vi "Main.vi"() -> ()   [LabVIEW 2023]
uses:
  Ctl/QMH Fundamentals - Message Cluster.ctl
  Ctl/Command.ctl
  Ctl/Global Parameter.ctl
  e830df23-c5e2-412d-a348-f1522410b5be.vi
  System.Speech
  3f4bac93-3011-4ff6-ad61-7a3954b40021.vi
panel:
  out "当前状态":string
  in  "Start?":bool
  out "识别结果 2":string caption="识别结果"
  out "灯 2":bool
  out "系统回复 2":string
  out "命令列表 2":string[](array[string])=["你好", "早上好", "中午好", "下午好", "分析", "测试", "音乐", "开灯", "关灯", "再见"] caption="命令列表"
  out "当前用户 2":string caption="当前用户"
  in  "LogOut 2":bool
  out "当前用户":string
  in  "LogOut":bool
  out "命令列表":string[](array[string])=["你好", "早上好", "中午好", "下午好", "分析", "测试", "音乐", "开灯", "关灯", "再见"]
  out "灯":bool
  out "系统回复":string
  out "识别结果":string
  # "基于声卡的语音识别与音频分析系统"
  # "基于声卡的语音识别与音频分析系统"
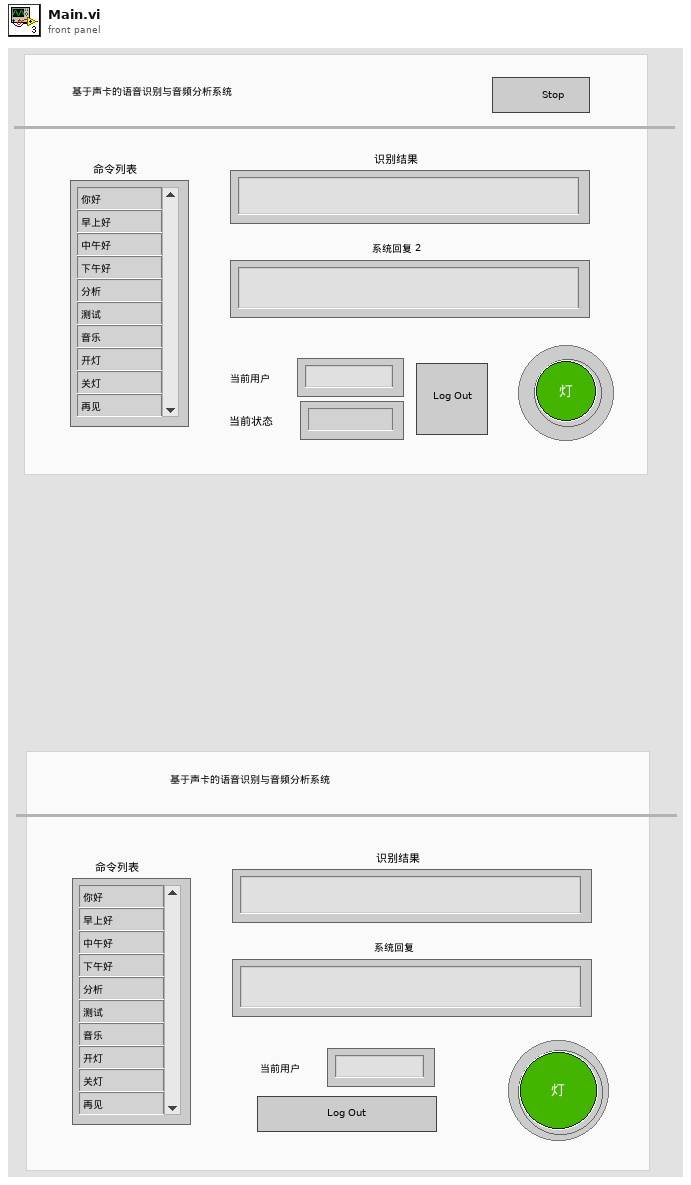
[diagram p1: front panel]
types:
  T1 = typedef "Command.ctl" = string[]
  T2 = typedef "Global Parameter.ctl" = cluster{"User Information":cluster{"用户名：":string, "密   码：":string}, "Login？":bool}
  T3 = typedef "QMH Fundamentals - Message Cluster.ctl" = cluster{"消息":string, "消息数据":variant}
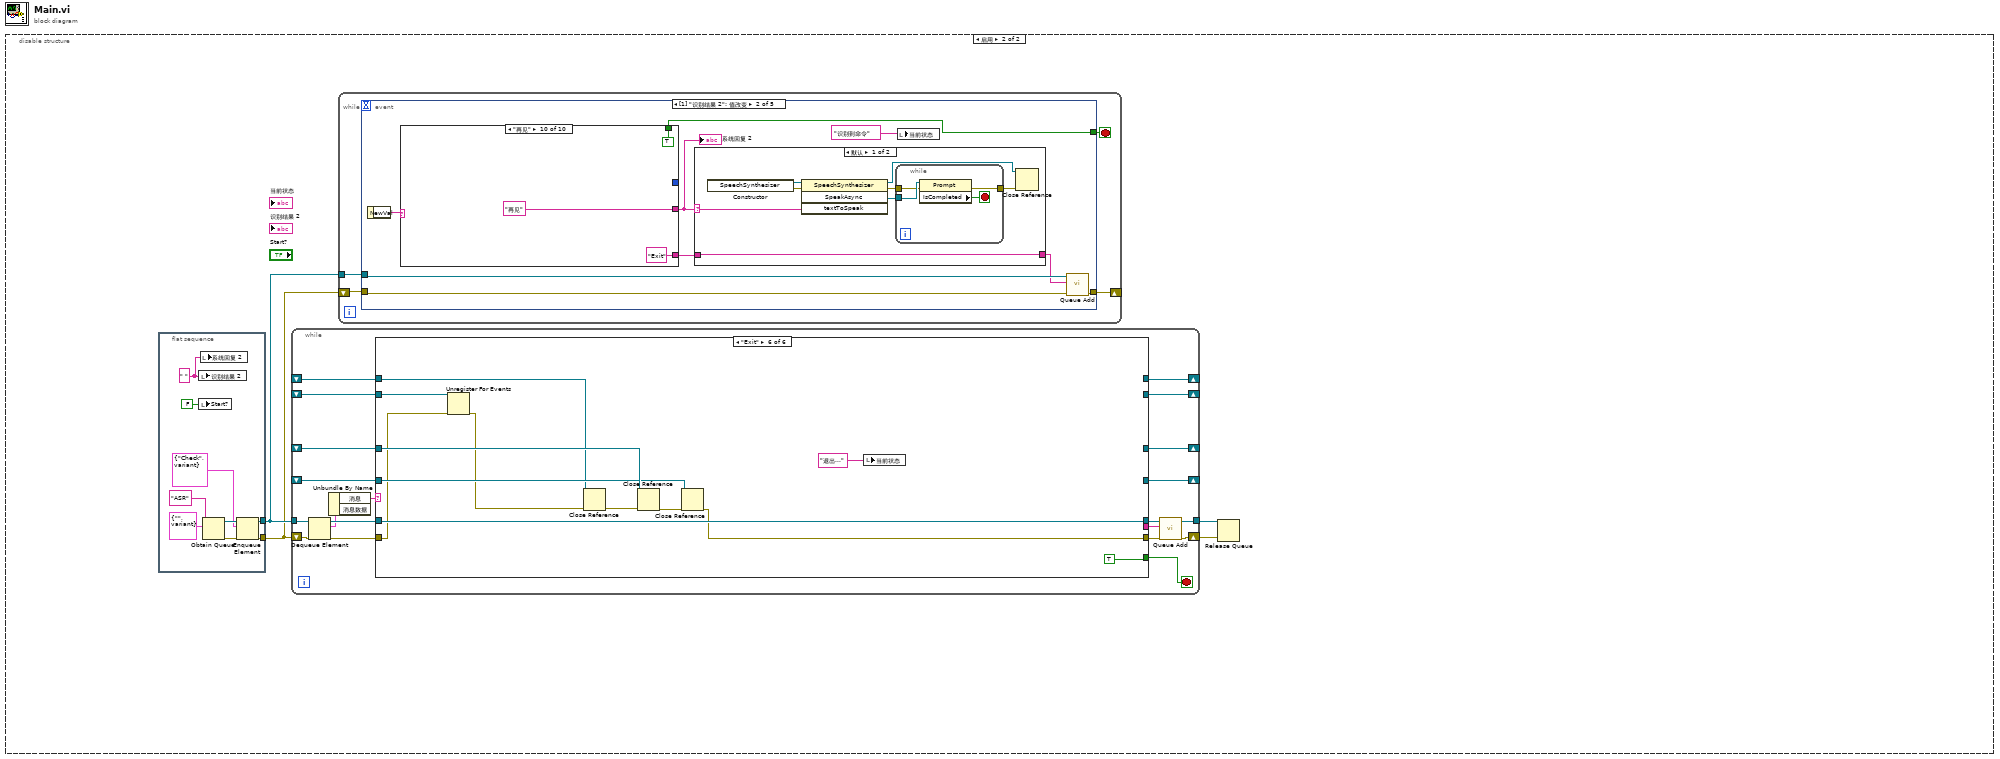
[diagram p0: block diagram]
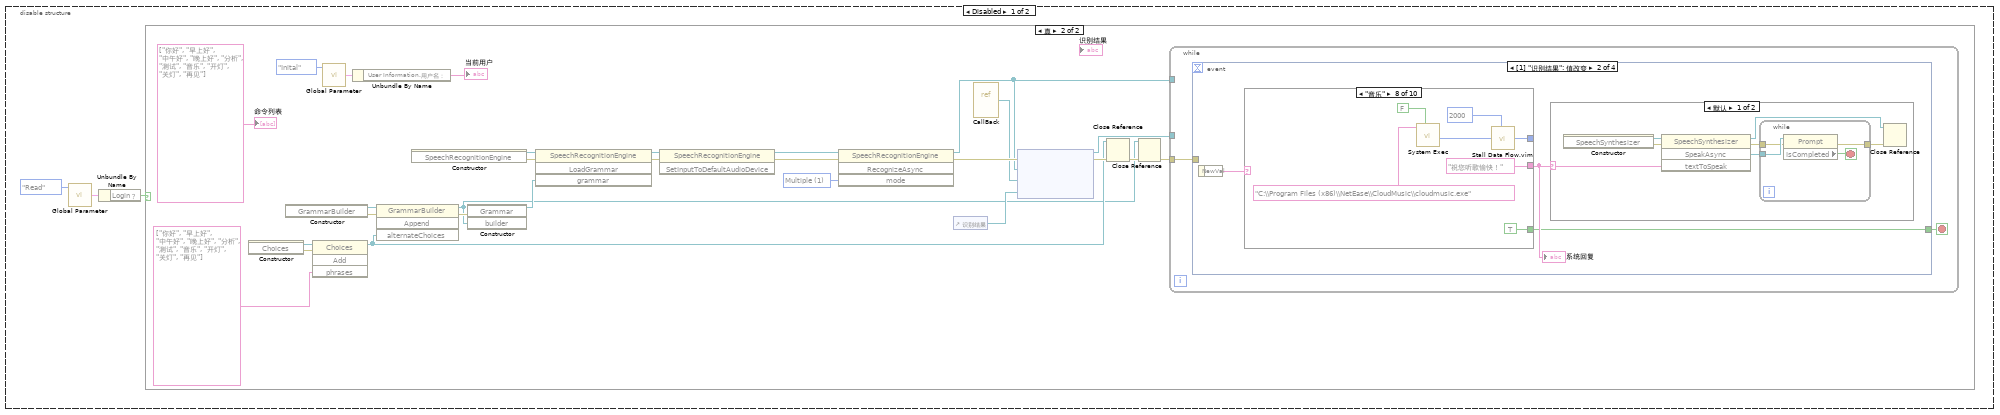
[diagram p2: hidden frame]
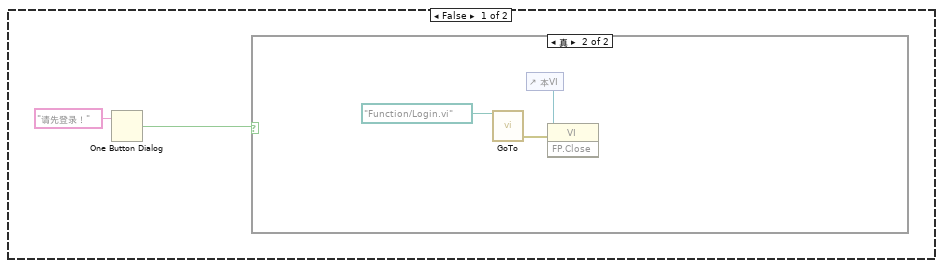
[diagram p3: hidden frame]
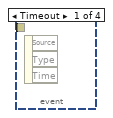
[diagram p5: hidden frame]
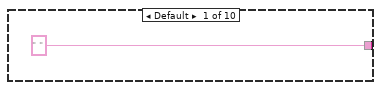
[diagram p7: hidden frame]
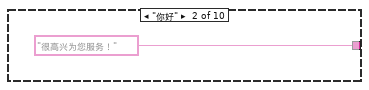
[diagram p8: hidden frame]
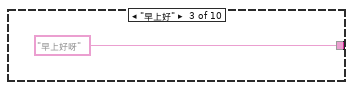
[diagram p9: hidden frame]
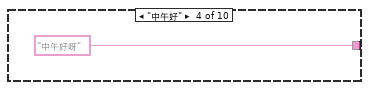
[diagram p10: hidden frame]
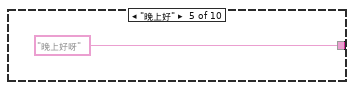
[diagram p11: hidden frame]
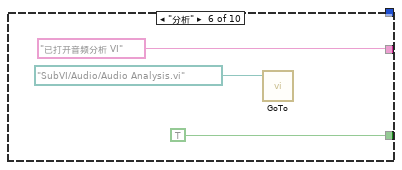
[diagram p12: hidden frame]
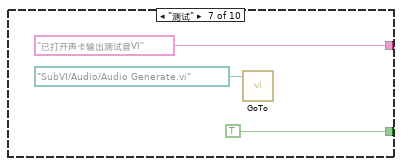
[diagram p13: hidden frame]
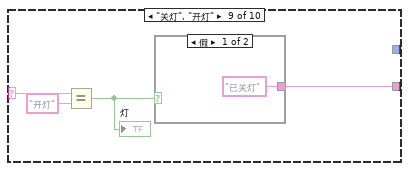
[diagram p14: hidden frame]
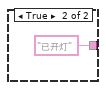
[diagram p15: hidden frame]
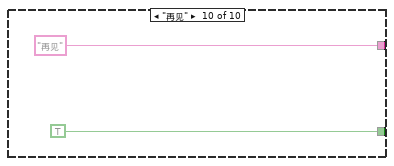
[diagram p16: hidden frame]
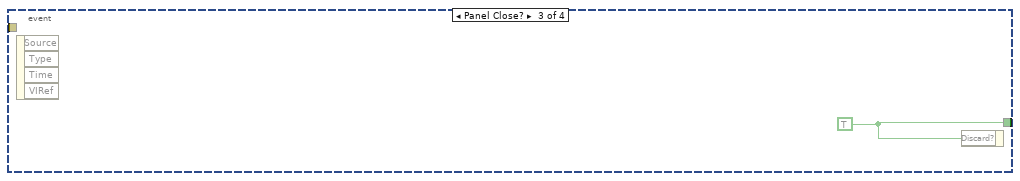
[diagram p17: hidden frame]
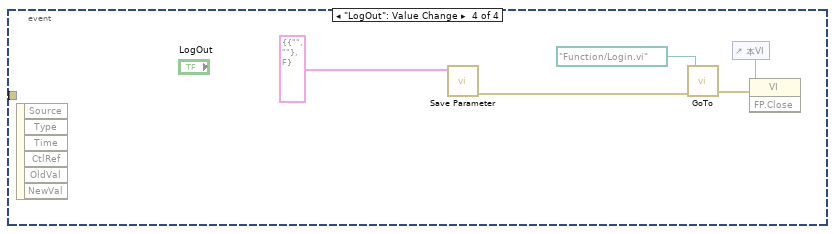
[diagram p18: hidden frame]
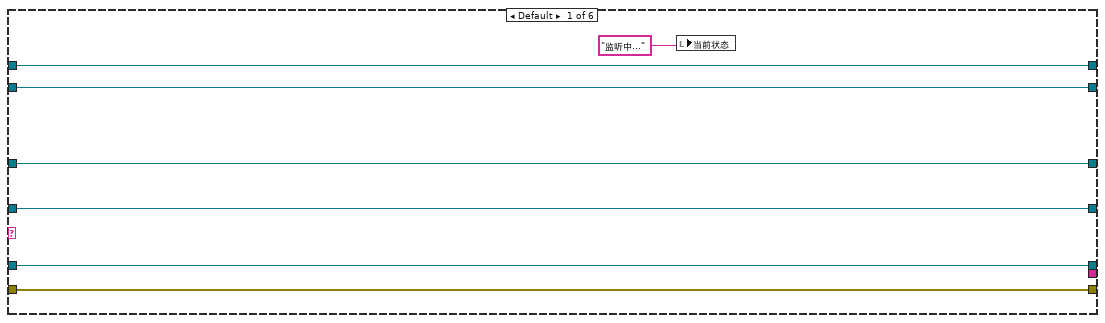
[diagram p19: hidden frame]
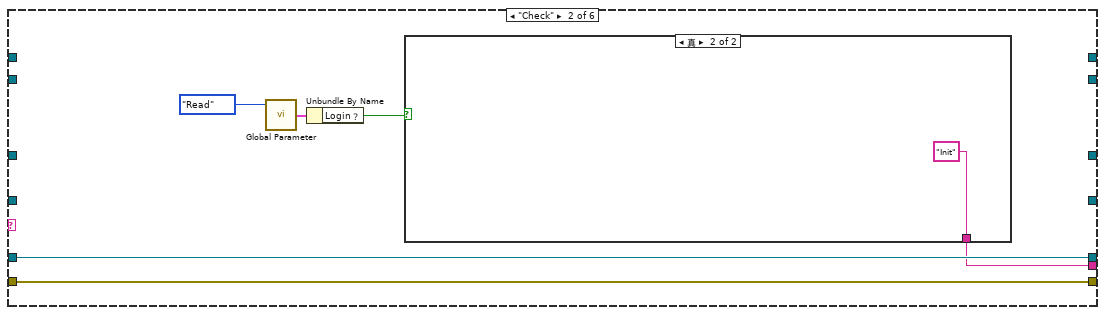
[diagram p20: hidden frame]
diagram:
  n1 = disable-structure shown="启用" {
    frame Disabled {
      n2 = call "Global Parameter.vi"("枚举"=enum16{"Inital", "Read", "Write", "Quit"}."Read") -> ("Read"=w2:T2)  [unwired: 3 in, 1 out]
      n3 = Unbundle By Name(w2) -> ("Login？"=w1:bool)
      n4 = case shown="真" w1 {
        frame False {
          n5 = One Button Dialog(message="请先登录！" ("消息")) -> (true=w4:bool)  [unwired: 1 in]
          n6 = case shown="真" w4 {
            frame False {
            }
            frame True {
              n7 = call "GoTo.vi"("名称或相对路径"=path "Function/Login.vi") -> ("错误输出"=w6:errorcluster)  [unwired: 4 in]
              n8 = control-ref of="本VI"() -> (w7:refnum<vi>)
              n9 = invoke class="VI" method="FP.Close"(reference=w7, error in=w6) -> ()  [unwired: 1 in, 3 out]
            }
          }
        }
        frame True {
          w29 = 1 items=["Single", "Multiple"] ("mode")
          n10 = constructor class="Choices"() -> (reference out=w35:refnum<k24>, error out=w28:errorcluster)  [unwired: 3 in, 1 out]
          n11 = constructor class="GrammarBuilder"() -> (reference out=w34:refnum<k24>, error out=w27:errorcluster)  [unwired: 3 in, 1 out]
          n12 = invoke on="调用节点" class="Choices" method="Add"(reference=w35, error in=w28, "phrases"=T1 ["你好", "早上好", "中午好", "晚上好", "分析", "测试", "音乐", "开灯", "关灯", "再见"]) -> (reference out=w18:refnum<k24>)  [unwired: 1 in, 3 out]
          n13 = call "Global Parameter.vi"("枚举"=enum16{"Inital", "Read", "Write", "Quit"}."Inital") -> ("Read"=w11:T2)  [unwired: 3 in, 1 out]
          n14 = Unbundle By Name(w11) -> ("User Information.用户名："=→"当前用户":string)
          n15 = invoke on="调用节点" class="GrammarBuilder" method="Append"(reference=w34, error in=w27, "alternateChoices"=w18) -> (reference out=w16:refnum<k24>, error out=w26:errorcluster)  [unwired: 1 in, 2 out]
          n16 = constructor class="SpeechRecognitionEngine"() -> (reference out=w33:refnum<k24>, error out=w25:errorcluster)  [unwired: 3 in, 1 out]
          n17 = constructor class="Grammar"(error in=w26, "builder"=w16) -> (reference out=w32:refnum<k24>)  [unwired: 2 in, 3 out]
          n18 = invoke on="调用节点" class="SpeechRecognitionEngine" method="LoadGrammar"(reference=w33, error in=w25, "grammar"=w32) -> (reference out=w31:refnum<k24>, error out=w24:errorcluster)  [unwired: 1 in, 2 out]
          n19 = invoke on="调用节点" class="SpeechRecognitionEngine" method="SetInputToDefaultAudioDevice"(reference=w31, error in=w24) -> (reference out=w30:refnum<k24>, error out=w23:errorcluster)  [unwired: 1 in, 1 out]
          n20 = invoke on="调用节点" class="SpeechRecognitionEngine" method="RecognizeAsync"(reference=w30, error in=w23, "mode"=w29) -> (reference out=w14:refnum<k24>, error out=w22:errorcluster)  [unwired: 1 in, 2 out]
          n21 = control-ref of="识别结果"() -> (w21:refnum<vi>)
          n22 = vi-ref "CallBack.vi"() -> ("vi reference"=w20:refnum<vi>)
          n23 = node(w22, w14, w20, w21) -> (w15:refnum<k27>, w19:errorcluster)  [unwired: 1 in]
          n24 = Close Reference(reference=w18, error in (no error)=w19) -> (error out=w17:errorcluster)
          n25 = Close Reference(reference=w16, error in (no error)=w17) -> (error out=w13:errorcluster)
          n26 = while {
            tunnel: w15 -> [_]
            tunnel: w14 -> [_]
            tunnel: w13 -> [w37]
            stop <- w38 stop-if-true
            n27 = event shown="[1] \"识别结果\": 值改变" {
              selector: _ -> [_ _ _ _]
              dyn-events: _ -> [_ _ _ _]
              timeout: _ -> [_ _ _ _]
              tunnel: [_ w39 w79 _] -> w38
              tunnel: w37 -> [_ _ _ _]
              event Timeout {
                n28 = event-data() -> ()  [unwired: 1 in, 3 out]
              }
              event "识别结果": Value Change {
                n29 = event-data() -> ("NewVal"=w41:string)  [unwired: 1 in]
                n30 = case shown="\"音乐\"" w41 {
                  selector: w41 -> [_ _ _ _ _ _ _ _ w74 _]
                  tunnel: [" " "很高兴为您服务！" "早上好呀" "中午好呀" "晚上好呀" "已打开音频分析 VI" "已打开声卡输出测试音VI" "祝您听歌愉快！" w72 "再见"] -> w40
                  tunnel: [_ _ _ _ _ _ _ w65 _ _] -> _
                  tunnel: [_ _ _ _ _ TRUE TRUE TRUE _ TRUE] -> w39
                  frame Default {
                  }
                  frame "你好" {
                  }
                  frame "早上好" {
                  }
                  frame "中午好" {
                  }
                  frame "晚上好" {
                  }
                  frame "分析" {
                    n31 = call "GoTo.vi"("名称或相对路径"=path "SubVI/Audio/Audio Analysis.vi") -> ()  [unwired: 4 in, 1 out]
                  }
                  frame "测试" {
                    n32 = call "GoTo.vi"("名称或相对路径"=path "SubVI/Audio/Audio Generate.vi") -> ()  [unwired: 4 in, 1 out]
                  }
                  frame "音乐" {
                    n33 = call <vilib>:"System Exec.vi"("wait until completion? (T)"=FALSE, "command line"="C:\\Program Files (x86)\\NetEase\\CloudMusic\\cloudmusic.exe") -> ("return code"=w68:i32)  [unwired: 6 in, 3 out]
                    n34 = call "Stall Data Flow.vim"("value in"=w68, "milliseconds to wait"=u32 2000) -> ("value out"=w65:i32)  [unwired: 1 out]
                  }
                  frame "关灯", "开灯" {
                    n35 = Equal?(x=w74, y="开灯") -> (x = y?=w71:bool)
                    "灯" <- w71
                    n36 = case shown="假" w71 {
                      tunnel: ["已关灯" "已开灯"] -> w72
                      frame False {
                      }
                      frame True {
                      }
                    }
                  }
                  frame "再见" {
                  }
                }
                "系统回复" <- w40
                n37 = case shown="默认" w40 {
                  selector: w40 -> [w48 _]
                  frame Default {
                    n38 = constructor class="SpeechSynthesizer"() -> (reference out=w43:refnum<k24>, error out=w47:errorcluster)  [unwired: 3 in, 1 out]
                    n39 = invoke on="调用节点" class="SpeechSynthesizer" method="SpeakAsync"(reference=w43, error in=w47, "textToSpeak"=w48) -> (reference out=w42:refnum<k24>, error out=w45:errorcluster, "SpeakAsync"=w46:refnum<k24>)  [unwired: 1 in, 1 out]
                    n40 = while {
                      tunnel: w46 -> [w52]
                      tunnel: w45 -> [w50]
                      tunnel: [w49] -> w44
                      stop <- w51 stop-if-true
                      n41 = property on="属性节点" class="Prompt"(reference=w52, error in=w50) -> (error out=w49:errorcluster, "IsCompleted"=w51:bool)  [unwired: 1 out]
                    }
                    n42 = Close Reference(reference=w42, error in (no error)=w44) -> ()  [unwired: 1 out]
                  }
                  frame " " {
                  }
                }
              }
              event Panel Close? {
                w79 = TRUE
                n43 = event-data() -> ()  [unwired: 1 in, 4 out]
                n44 = event-data("Discard?"=w79) -> ()  [unwired: 1 in, 1 out]
              }
              event "LogOut": Value Change {
                n45 = event-data() -> ()  [unwired: 1 in, 6 out]
                n46 = call "Save Parameter.vi"("Parameter In"=T2 {"User Information"={"用户名："="", "密   码："=""}, "Login？"=FALSE} ("Write")) -> ("error out"=w80:errorcluster)  [unwired: 10 in]
                n47 = call "GoTo.vi"("错误输入（无错误）"=w80, "名称或相对路径"=path "Function/Login.vi") -> ("错误输出"=w82:errorcluster)  [unwired: 3 in]
                n48 = control-ref of="本VI"() -> (w83:refnum<vi>)
                n49 = invoke class="VI" method="FP.Close"(reference=w83, error in=w82) -> ()  [unwired: 1 in, 3 out]
              }
            }
          }
          "命令列表" <- T1 ["你好", "早上好", "中午好", "晚上好", "分析", "测试", "音乐", "开灯", "关灯", "再见"] ("phrases")
        }
      }
    }
    frame Enabled {
      n50 = flat-sequence {
        tunnel: [w92] -> w88
        tunnel: [w91] -> w87
        frame #0 {
          w90 = " " ("识别结果 2")
          n51 = local write "识别结果 2"(w90) -> ()
          n52 = local write "Start?"(FALSE ("Start?")) -> ()
          n53 = local write "系统回复 2"(w90) -> ()
          n54 = Obtain Queue(name (unnamed)="ASR" ("名称（未命名）"), element data type=T3 {"消息"="", "消息数据"=variant} ("Message Cluster")) -> (queue out=w95:refnum<queue>, error out=w96:errorcluster)  [unwired: 3 in, 1 out]
          n55 = Enqueue Element(queue=w95, element=T3 {"消息"="Check", "消息数据"=variant} ("元素"), error in (no error)=w96) -> (queue out=w92:refnum<queue>, error out=w91:errorcluster)  [unwired: 1 in, 1 out]
        }
      }
      n56 = while {
        shift-right: [w105] -> w86
        shift-left: w87 -> [w117]
        tunnel: w88 -> [w116]
        shift-right: [w112] -> _
        shift-left: _ -> [w101]
        shift-right: [w111] -> _
        shift-left: _ -> [w102]
        shift-right: [w110] -> _
        shift-left: _ -> [w109]
        shift-right: [w108] -> _
        shift-left: _ -> [w103]
        tunnel: [w106] -> w85
        stop <- w100 stop-if-true
        n57 = Dequeue Element(queue=w116, error in (no error)=w117) -> (queue out=w115:refnum<queue>, element=w114:T3, error out=w99:errorcluster)  [unwired: 1 in, 1 out]
        n58 = Unbundle By Name(w114) -> ("消息"=w113:string)  [unwired: 1 out]
        n59 = case shown="\"Exit\"" w113 {
          tunnel: w115 -> [w124 w130 w161 w171 w180 w192]
          tunnel: [w124 w130 w161 w171 w180 w192] -> w107
          tunnel: [w120 _ w149 w166 w176 _] -> w112
          tunnel: [w121 _ w148 w167 w177 _] -> w111
          tunnel: [w123 _ w145 w168 w178 _] -> w110
          tunnel: w109 -> [w123 _ _ w169 w179 w185]
          tunnel: [w122 _ w144 w165 w175 _] -> w108
          tunnel: [_ w126 _ _ _ _] -> w104
          tunnel: w103 -> [w122 _ _ w165 w175 w190]
          tunnel: w102 -> [w121 _ _ w167 w177 w189]
          tunnel: w101 -> [w120 _ _ w166 w176 w188]
          tunnel: [_ _ _ _ _ TRUE] -> w100
          tunnel: w99 -> [w119 w125 w139 w164 w174 w182]
          tunnel: [w119 w125 w139 w163 w173 w183] -> w98
          frame Default {
            n60 = local write "当前状态"("监听中..." ("当前状态")) -> ()
          }
          frame "Check" {
            n61 = call "Global Parameter.vi"("枚举"=enum16{"Inital", "Read", "Write", "Quit"}."Read") -> ("Read"=w129:T2)  [unwired: 3 in, 1 out]
            n62 = Unbundle By Name(w129) -> ("Login？"=w127:bool)
            n63 = case shown="真" w127 {
              tunnel: ["Check" ("消息") "Init" ("消息")] -> w126
              frame False {
                n64 = One Button Dialog(message="请先登录！" ("消息")) -> (true=w132:bool)  [unwired: 1 in]
                n65 = case shown="假" w132 {
                  frame False {
                  }
                  frame True {
                    n66 = call "GoTo.vi"("名称或相对路径"=path "Function/Login.vi") -> ("错误输出"=w134:errorcluster)  [unwired: 4 in]
                    n67 = control-ref of="本VI"() -> (w135:refnum<vi>)
                    n68 = invoke class="VI" method="FP.Close"(reference=w135, error in=w134) -> ()  [unwired: 1 in, 3 out]
                  }
                }
              }
              frame True {
              }
            }
          }
          frame "Init" {
            w150 = T1 ["你好", "早上好", "中午好", "晚上好", "分析", "测试", "音乐", "开灯", "关灯", "再见"] ("phrases")
            n69 = constructor class="Choices"() -> (reference out=w160:refnum<k24>, error out=w155:errorcluster)  [unwired: 3 in, 1 out]
            n70 = call "Global Parameter.vi"("枚举"=enum16{"Inital", "Read", "Write", "Quit"}."Inital") -> ("Read"=w143:T2)  [unwired: 3 in, 1 out]
            n71 = constructor class="GrammarBuilder"() -> (reference out=w159:refnum<k24>, error out=w154:errorcluster)  [unwired: 3 in, 1 out]
            n72 = Unbundle By Name(w143) -> ("User Information.用户名："=→"当前用户 2":string)
            n73 = invoke on="调用节点" class="Choices" method="Add"(reference=w160, error in=w155, "phrases"=w150) -> (reference out=w149:refnum<k24>)  [unwired: 1 in, 3 out]
            n74 = invoke on="调用节点" class="GrammarBuilder" method="Append"(reference=w159, error in=w154, "alternateChoices"=w149) -> (reference out=w148:refnum<k24>, error out=w153:errorcluster)  [unwired: 1 in, 2 out]
            n75 = constructor class="SpeechRecognitionEngine"() -> (reference out=w158:refnum<k24>, error out=w152:errorcluster)  [unwired: 3 in, 1 out]
            n76 = constructor class="Grammar"(error in=w153, "builder"=w148) -> (reference out=w157:refnum<k24>)  [unwired: 2 in, 3 out]
            n77 = invoke on="调用节点" class="SpeechRecognitionEngine" method="LoadGrammar"(reference=w158, error in=w152, "grammar"=w157) -> (reference out=w156:refnum<k24>, error out=w151:errorcluster)  [unwired: 1 in, 2 out]
            n78 = invoke on="调用节点" class="SpeechRecognitionEngine" method="SetInputToDefaultAudioDevice"(reference=w156, error in=w151) -> (reference out=w145:refnum<k24>, error out=w140:errorcluster)  [unwired: 1 in, 1 out]
            n79 = local write "当前状态"("待开始" ("当前状态")) -> ()
            n80 = control-ref of="识别结果 2"() -> (w146:refnum<vi>)
            n81 = vi-ref "CallBack.vi"() -> ("vi reference"=w147:refnum<vi>)
            n82 = node(w140, w145, w147, w146) -> (w144:refnum<k27>)  [unwired: 1 in, 1 out]
            "命令列表 2" <- w150
          }
          frame "Start" {
            w170 = 1 items=["Single", "Multiple"] ("mode")
            n83 = invoke on="调用节点" class="SpeechRecognitionEngine" method="RecognizeAsync"(reference=w169, error in=w164, "mode"=w170) -> (reference out=w168:refnum<k24>, error out=w163:errorcluster)  [unwired: 1 in, 2 out]
            n84 = local write "当前状态"("监听中..." ("当前状态")) -> ()
          }
          frame "Stop" {
            n85 = invoke on="调用节点" class="SpeechRecognitionEngine" method="RecognizeAsyncStop"(reference=w179, error in=w174) -> (reference out=w178:refnum<k24>, error out=w173:errorcluster)  [unwired: 1 in, 1 out]
            n86 = local write "当前状态"("已停止" ("当前状态")) -> ()
          }
          frame "Exit" {
            n87 = Unregister For Events(event registration refnum=w190, error in=w182) -> (error out=w187:errorcluster)
            n88 = Close Reference(reference=w185, error in (no error)=w187) -> (error out=w186:errorcluster)
            n89 = Close Reference(reference=w189, error in (no error)=w186) -> (error out=w191:errorcluster)
            n90 = Close Reference(reference=w188, error in (no error)=w191) -> (error out=w183:errorcluster)
            n91 = local write "当前状态"("退出..." ("当前状态")) -> ()
          }
        }
        n92 = call "Queue Add.vi"("错误输入（无错误）"=w98, "消息"=w104, "队列输入"=w107) -> ("错误输出"=w105:errorcluster, "队列输出"=w106:refnum<queue>)  [unwired: 7 in]
      }
      n93 = while {
        tunnel: w88 -> [w195]
        shift-right: [w193] -> _
        shift-left: w87 -> [w194]
        stop <- w196 stop-if-true
        n94 = event shown="[1] \"识别结果 2\": 值改变" {
          selector: _ -> [_ _ _ _ _]
          dyn-events: _ -> [_ _ _ _ _]
          timeout: _ -> [_ _ _ _ _]
          tunnel: [_ w198 _ w265 TRUE] -> w196
          tunnel: w195 -> [_ w206 w251 w264 w272]
          tunnel: w194 -> [w197 w205 w250 w263 w270]
          tunnel: [w197 w204 w249 w261 w266] -> w193
          event Timeout {
            n95 = event-data() -> ()  [unwired: 1 in, 3 out]
          }
          event "识别结果 2": Value Change {
            n96 = event-data() -> ("NewVal"=w201:string)  [unwired: 1 in]
            n97 = case shown="\"再见\"" w201 {
              selector: w201 -> [_ _ _ _ _ _ _ _ w243 _]
              tunnel: [" " "很高兴为您服务！" "早上好呀" "中午好呀" "晚上好呀" "已打开音频分析 VI" "已打开声卡输出测试音VI" "祝您听歌愉快！" w241 "再见"] -> w203
              tunnel: [_ _ _ _ _ _ _ w234 _ _] -> _
              tunnel: [_ _ _ _ _ "Exit" ("消息") "Exit" ("消息") "Exit" ("消息") _ "Exit" ("消息")] -> w202
              tunnel: [_ _ _ _ _ TRUE TRUE TRUE _ TRUE] -> w198
              frame Default {
              }
              frame "你好" {
              }
              frame "早上好" {
              }
              frame "中午好" {
              }
              frame "晚上好" {
              }
              frame "分析" {
                n98 = call "GoTo.vi"("名称或相对路径"=path "SubVI/Audio/Audio Analysis.vi") -> ()  [unwired: 4 in, 1 out]
              }
              frame "测试" {
                n99 = call "GoTo.vi"("名称或相对路径"=path "SubVI/Audio/Audio Generate.vi") -> ()  [unwired: 4 in, 1 out]
              }
              frame "音乐" {
                n100 = call <vilib>:"System Exec.vi"("wait until completion? (T)"=FALSE, "command line"="C:\\Program Files (x86)\\NetEase\\CloudMusic\\cloudmusic.exe") -> ("return code"=w237:i32)  [unwired: 6 in, 3 out]
                n101 = call "Stall Data Flow.vim"("value in"=w237, "milliseconds to wait"=u32 2000) -> ("value out"=w234:i32)  [unwired: 1 out]
              }
              frame "关灯", "开灯" {
                n102 = Equal?(x=w243, y="开灯") -> (x = y?=w240:bool)
                "灯 2" <- w240
                n103 = case shown="假" w240 {
                  tunnel: ["已关灯" "已开灯"] -> w241
                  frame False {
                  }
                  frame True {
                  }
                }
              }
              frame "再见" {
              }
            }
            "系统回复 2" <- w203
            n104 = case shown="默认" w203 {
              selector: w203 -> [w214 _]
              tunnel: w202 -> [w207 _]
              tunnel: [w207 _] -> w200
              frame Default {
                n105 = constructor class="SpeechSynthesizer"() -> (reference out=w209:refnum<k24>, error out=w213:errorcluster)  [unwired: 3 in, 1 out]
                n106 = invoke on="调用节点" class="SpeechSynthesizer" method="SpeakAsync"(reference=w209, error in=w213, "textToSpeak"=w214) -> (reference out=w208:refnum<k24>, error out=w211:errorcluster, "SpeakAsync"=w212:refnum<k24>)  [unwired: 1 in, 1 out]
                n107 = while {
                  tunnel: w212 -> [w218]
                  tunnel: w211 -> [w216]
                  tunnel: [w215] -> w210
                  stop <- w217 stop-if-true
                  n108 = property on="属性节点" class="Prompt"(reference=w218, error in=w216) -> (error out=w215:errorcluster, "IsCompleted"=w217:bool)  [unwired: 1 out]
                }
                n109 = Close Reference(reference=w208, error in (no error)=w210) -> ()  [unwired: 1 out]
              }
              frame " " {
              }
            }
            n110 = local write "当前状态"("识别到命令" ("当前状态")) -> ()
            n111 = call "Queue Add.vi"("错误输入（无错误）"=w205, "消息"=w200, "队列输入"=w206) -> ("错误输出"=w204:errorcluster)  [unwired: 7 in, 1 out]
          }
          event "Start?": Value Change {
            n112 = event-data() -> ("NewVal"=w252:bool)  [unwired: 1 in]
            n113 = case shown="假" w252 {
              tunnel: w251 -> [w255 w260]
              tunnel: w250 -> [w254 w259]
              tunnel: [w253 w257] -> w249
              frame False {
                n114 = call "Queue Add.vi"("错误输入（无错误）"=w254, "消息"="Stop", "队列输入"=w255) -> ("错误输出"=w253:errorcluster)  [unwired: 7 in, 1 out]
              }
              frame True {
                n115 = call "Queue Add.vi"("错误输入（无错误）"=w259, "消息"="Start", "队列输入"=w260) -> ("错误输出"=w257:errorcluster)  [unwired: 7 in, 1 out]
              }
            }
          }
          event Panel Close? {
            w265 = TRUE
            n116 = event-data() -> ()  [unwired: 1 in, 4 out]
            n117 = call "Queue Add.vi"("错误输入（无错误）"=w263, "消息"="Exit", "队列输入"=w264) -> ("错误输出"=w261:errorcluster)  [unwired: 7 in, 1 out]
            n118 = event-data("Discard?"=w265) -> ()  [unwired: 1 in, 1 out]
          }
          event "LogOut 2": Value Change {
            n119 = event-data() -> ()  [unwired: 1 in, 1 out]
            n120 = call "Queue Add.vi"("错误输入（无错误）"=w270, "消息"="Exit", "队列输入"=w272) -> ("错误输出"=w266:errorcluster)  [unwired: 7 in, 1 out]
            n121 = call "Save Parameter.vi"("Parameter In"=T2 {"User Information"={"用户名："="", "密   码："=""}, "Login？"=FALSE} ("Write")) -> ("error out"=w268:errorcluster)  [unwired: 10 in]
            n122 = call "GoTo.vi"("错误输入（无错误）"=w268, "名称或相对路径"=path "Function/Login.vi") -> ()  [unwired: 3 in, 1 out]
          }
        }
      }
      n123 = Release Queue(queue=w85, error in (no error)=w86) -> ()  [unwired: 1 in, 3 out]
    }
  }
